vi "初始化使用次数和寿命的界面.vi"(11 "VISA  2":refnum<visa-resource-name>="COM3") -> ()   [LabVIEW 2011]
panel:
  in  "Init_Exit":bool=TRUE
  in  "Init_Start":bool=TRUE
  out "无符号字节数组":u8[](array[numeric]) format="%.0x"
  out "result":bool
  in  "开始截取位":i32=1
  out "Data Out":u8[](array[numeric])
  in  "截取长度":i32=2
  in  "输入数组":i32[](array[numeric])=[238, 0, 21, 0, 1, 128, 5, 8, 18, 52, 86, 120, 85, 7, 208, 238, 169, 255, 252, 255, 255] format="%.0x"
  # "初始化使用次数和设置使用寿命"
  # "3.初始化计数模块的已经使用次数和可以使用的使用寿命。（写操作）\nEE 00 15 00 01 80 05 08 12 34 56 78 55 00 10 EE A9 FF FC FF FF\n命令解释：\n0x05-0x08 可读写区域，写入0x12,0x34,0x56,0x78后测试板记录使用次数将清空；\n命令解释：\n0x09-0x0C 可读写区域，用于修改预设测试板的使用寿命，其中0x09位必须是0x55,0x0C位必须是0xEE，0x0A-0x0B表示要写入的预设值。（高位在前，低位在后）\n返回信息如下：\nEE 00 11 00 00 80 00 04 00 00 00 10 85 FF FC FF FF"
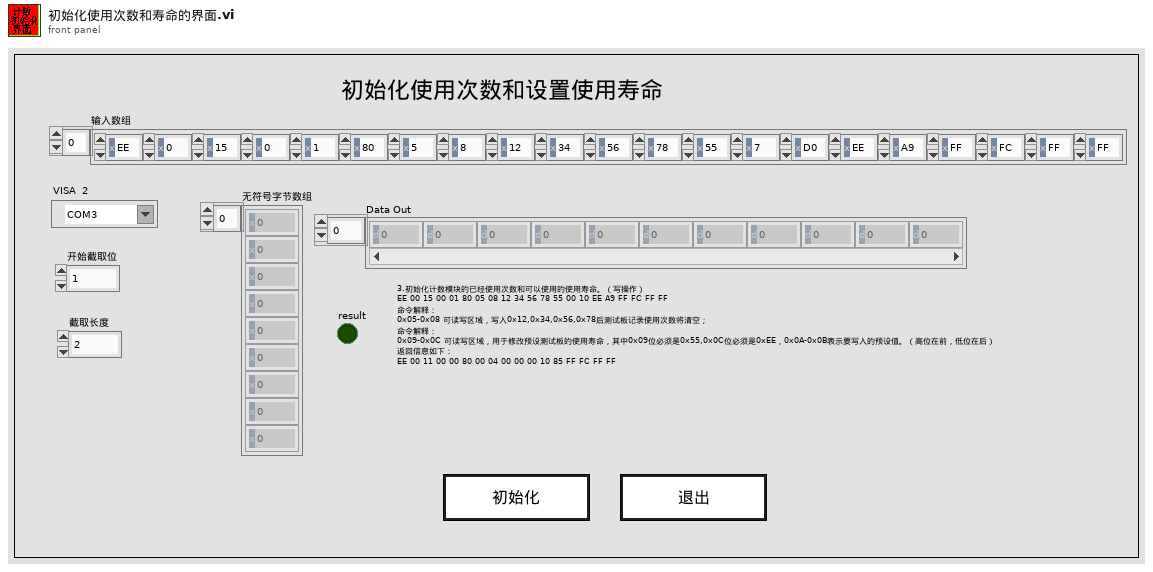
[diagram p1: front panel]
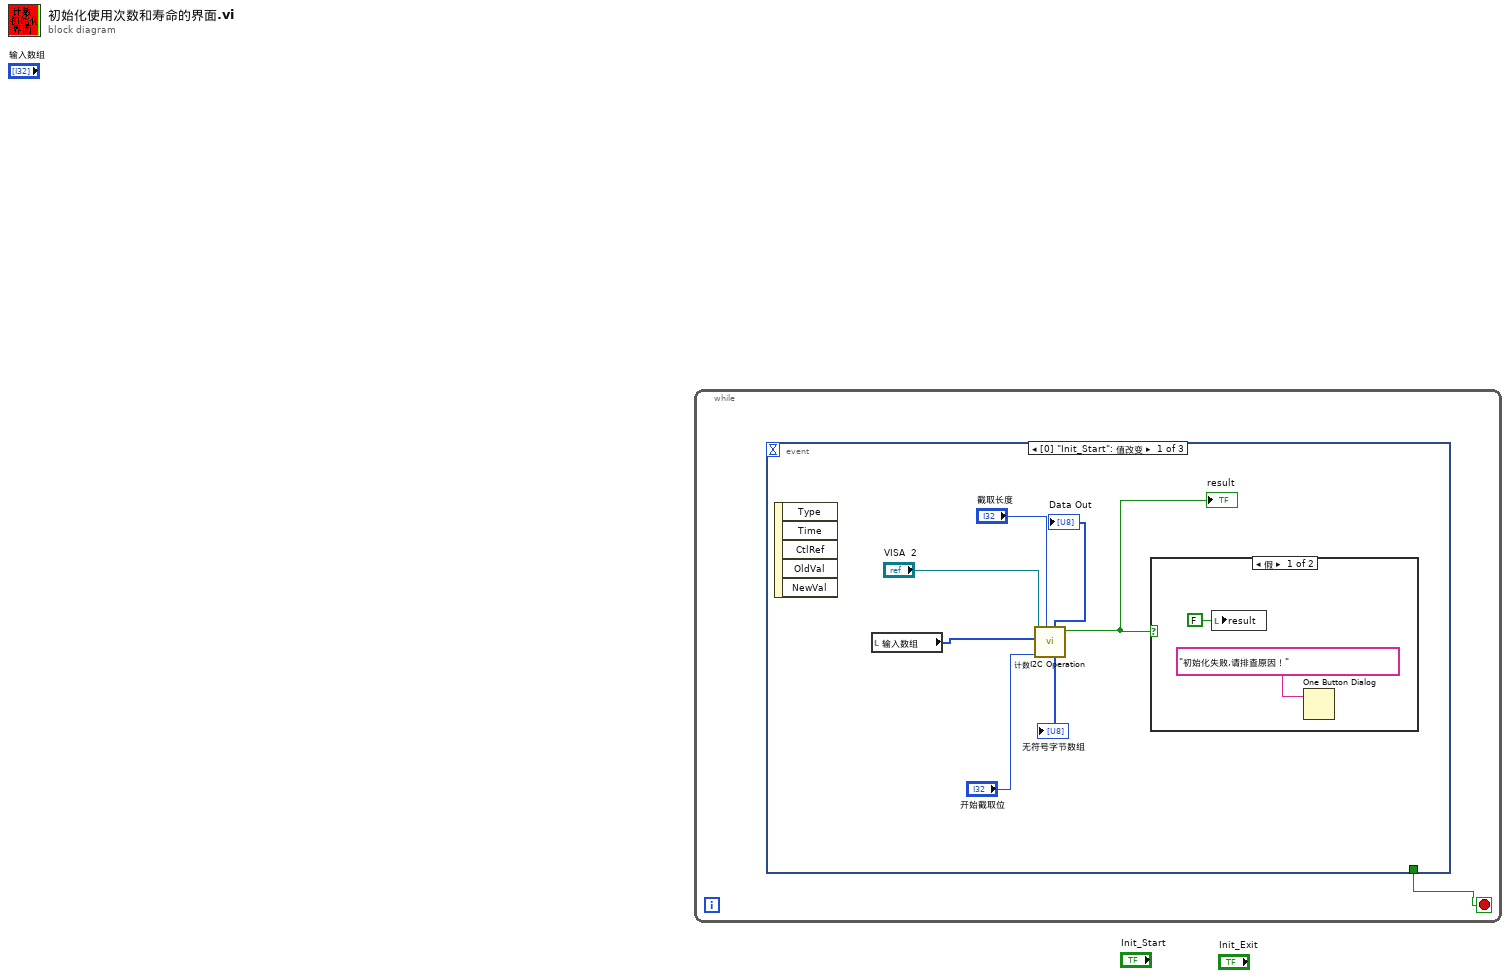
[diagram p0: block diagram]
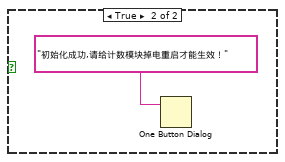
[diagram p2: hidden frame]
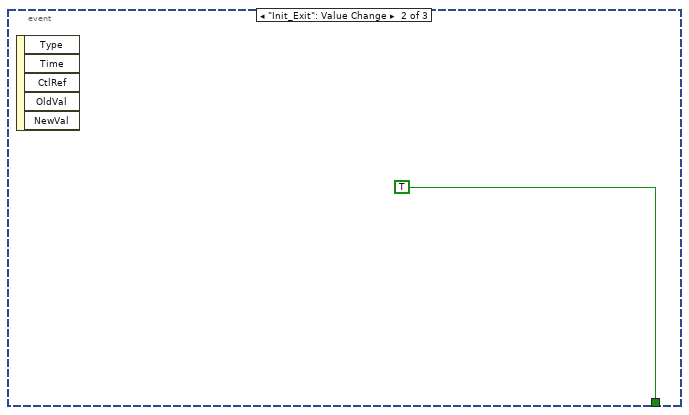
[diagram p3: hidden frame]
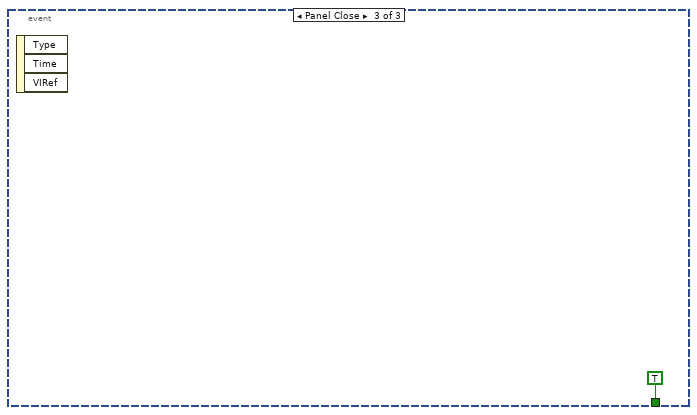
[diagram p4: hidden frame]
diagram:
  n1 = while {
    stop <- w1 stop-if-true
    n2 = event shown="[0] \"Init_Start\": 值改变" {
      selector: _ -> [_ _ _]
      dyn-events: _ -> [_ _ _]
      timeout: _ -> [_ _ _]
      tunnel: [_ TRUE TRUE] -> w1
      event "Init_Start": Value Change {
        n3 = event-data() -> ()  [unwired: 1 in, 5 out]
        n4 = local read "输入数组"() -> (w8:i32[])
        n5 = call "计数I2C Operation.vi"("截取长度"="截取长度", "开始截取位"="开始截取位", "输入数组"=w8, "VISA  2"="VISA  2") -> ("result"=w2:bool, "无符号字节数组"=→"无符号字节数组":u8[], "Data Out"=→"Data Out":u8[])  [unwired: 5 in]
        "result" <- w2
        n6 = case shown="假" w2 {
          frame False {
            n7 = local write "result"(FALSE ("result")) -> ()
            n8 = One Button Dialog(message="初始化失败,请排查原因！" ("消息")) -> ()  [unwired: 1 in, 1 out]
          }
          frame True {
            n9 = One Button Dialog(message="初始化成功,请给计数模块掉电重启才能生效！" ("消息")) -> ()  [unwired: 1 in, 1 out]
          }
        }
      }
      event "Init_Exit": Value Change {
        n10 = event-data() -> ()  [unwired: 1 in, 5 out]
      }
      event Panel Close {
        n11 = event-data() -> ()  [unwired: 1 in, 3 out]
      }
    }
  }
